vi "LOG.vi"(1 "I":dbl, 2 "N":dbl, 3 "END":dbl, 4 "INITIAL":dbl) -> (0 "数值":dbl)   [LabVIEW 2017]
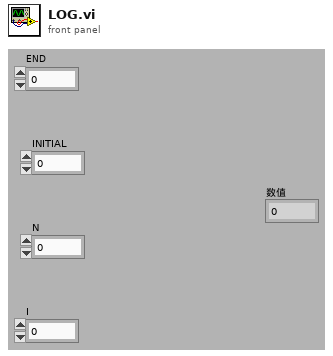
[diagram p1: front panel]
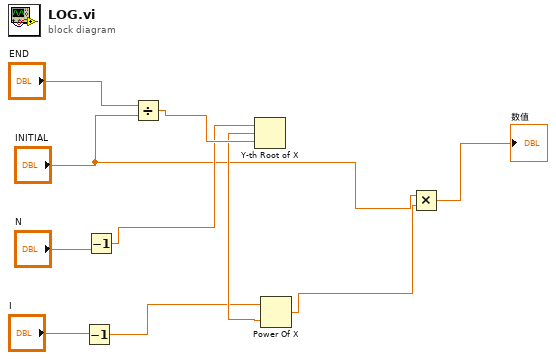
[diagram p0: block diagram]
diagram:
  n1 = Decrement(x="I") -> (x-1=w4:dbl)
  n2 = Decrement(x="N") -> (x-1=w7:dbl)
  n3 = Divide(x="END", y="INITIAL") -> (x/y=w8:dbl)
  n4 = Y-th Root of X(1:w8, 2:w7) -> (0:w5:dbl)
  n5 = Power Of X(1:w5, 2:w4) -> (0:w2:dbl)
  n6 = Multiply(x="INITIAL", y=w2) -> (x*y=→"数值":dbl)
